vi "SubVI Tester.vi"() -> ()   [LabVIEW 2012]
panel:
  out "警告文本":string="无警告"
  out "警告？":bool
  out "温度计":dbl(slide) scale=0.0..100.0
  in  "最低温度":dbl=10.0
  in  "最高温度":dbl=30.0
  in  "停止":bool
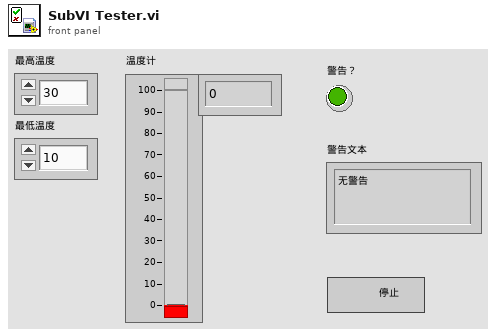
[diagram p1: front panel]
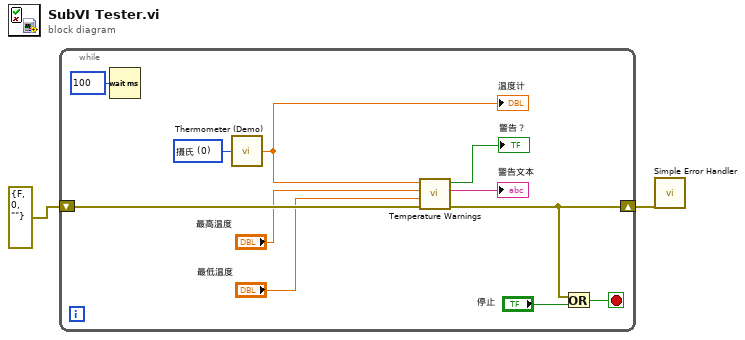
[diagram p0: block diagram]
diagram:
  n1 = while {
    shift-right: [w9] -> w2
    shift-left: cluster{"状态":bool, "代码":i32, "源":string} {"状态"=FALSE, "代码"=0, "源"=""} ("错误输出") -> [w10]
    stop <- w11 stop-if-true
    w3 = u16 0 items=["摄氏", "华氏"] ("单位（0：摄氏度）")
    n2 = Wait (ms) ("等待(ms)")(milliseconds to wait=u32 100 ("等待时间（毫秒）")) -> ()  [unwired: 1 out]
    n3 = call "Thermometer (Demo).vi"("单位（0：摄氏度）"=w3) -> ("温度值"=w8:dbl)
    "温度计" <- w8
    n4 = call "Temperature Warnings.vi"("错误输入"=w10, "最低温度"="最低温度", "最高温度"="最高温度", "当前温度"=w8) -> ("错误输出"=w9:cluster{"状态":bool, "代码":i32, "源":string}, "警告文本"=→"警告文本":string, "警告？"=→"警告？":bool)  [unwired: 5 in]
    n5 = Or ("或")(x=w9, y="停止") -> (x .or. y?=w11:bool)
  }
  n6 = call <vilib>:"Simple Error Handler.vi"("error in (no error)"=w2) -> ()  [unwired: 4 in, 5 out]
